vi "HTMLURLEncoding.vi"(11 "InputString":string) -> (3 "URLEncodedString":string)   [LabVIEW 2019]
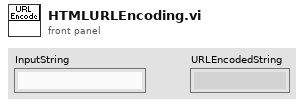
[diagram p1: front panel]
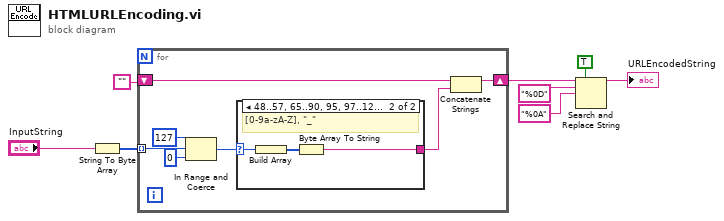
[diagram p0: block diagram]
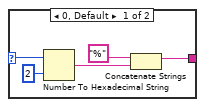
[diagram p2: hidden frame]
diagram:
  n1 = String To Byte Array(string="InputString") -> (unsigned byte array=w1:u8[])
  n2 = for {
    tunnel: w1 -> [w12] mode=indexing
    shift-right: [w13] -> w7
    shift-left: "" -> [w14]
    n3 = In Range and Coerce(upper limit=u8 127, x=w12, lower limit=u8 0) -> (coerced(x)=w11:u8)  [unwired: 1 out]
    n4 = case shown="48..57, 65..90, 95, 97..122" w11 {
      selector: w11 -> [w20 w23]
      tunnel: [w16 w21] -> w15
      frame 0, Default {
        n5 = Number To Hexadecimal String(1:i16 2 ("width (-)"), 2:w20) -> (0:w18:string)
        n6 = Concatenate Strings("%" ("string"), w18) -> (w16:string)
      }
      frame 48..57, 65..90, 95, 97..122 {
        # "[0-9a-zA-Z], \"_\""
        n7 = Build Array(w23) -> (w22:u8[])
        n8 = Byte Array To String(unsigned byte array=w22) -> (string=w21:string)
      }
    }
    n9 = Concatenate Strings(w14, w15) -> (w13:string)
  }
  n10 = Search and Replace String(replace all?=TRUE ("replace all? (F)"), input string=w7, search string="%0D", replace string="%0A" ("replace string (\"\")")) -> (result string=→"URLEncodedString":string)  [unwired: 4 in, 3 out]
